vi "Set File to Run as Admin.vi"(8 "Error In":errorcluster, 11 "Path to file that needs to be run as admin":path) -> (0 "Error Out":errorcluster)   [LabVIEW 2014]
panel:
  in  "working directory":path=path ""
  out "concatenated string":string
  out "standard error":string
  out "standard output":string
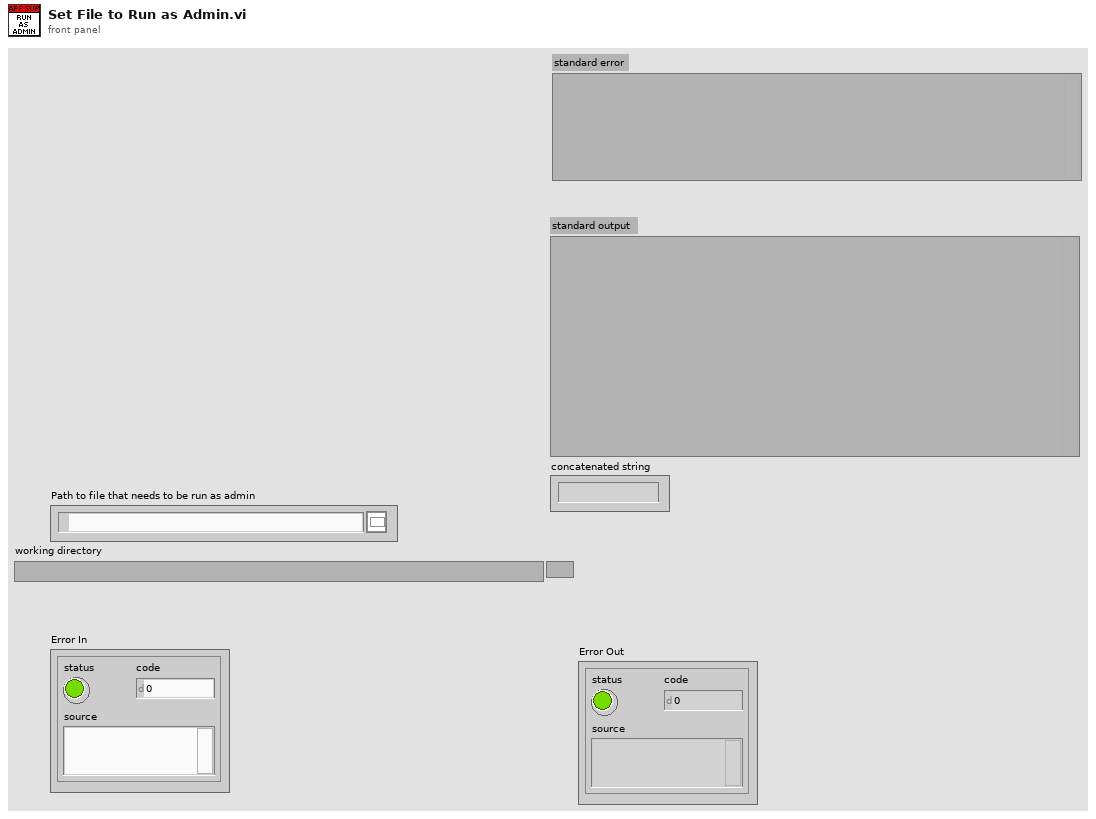
[diagram p1: front panel]
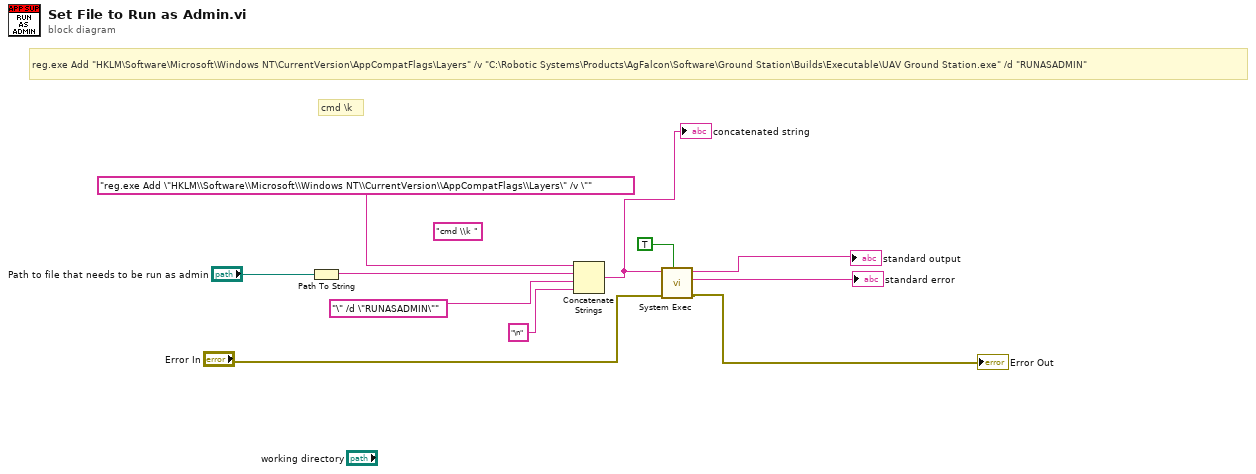
[diagram p0: block diagram]
diagram:
  (unwired) "cmd \\k " ("command line")
  # "cmd \\k"
  # "reg.exe Add \"HKLM\\Software\\Microsoft\\Windows NT\\CurrentVersion\\AppCompatFlags\\Layers\" /v \"C:\\Robotic Systems\\Products\\AgFalcon\\Software\\Ground Station\\Builds\\Executable\\UAV Ground Station.exe\" /d \"RUNASADMIN\""
  n1 = Path To String(path="Path to file that needs to be run as admin") -> (string=w9:string)
  n2 = Concatenate Strings("reg.exe Add \"HKLM\\Software\\Microsoft\\Windows NT\\CurrentVersion\\AppCompatFlags\\Layers\" /v \"" ("command line"), w9, "\" /d \"RUNASADMIN\"" ("command line"), "\n") -> (w2:string)
  "concatenated string" <- w2
  n3 = call <vilib>:"System Exec.vi"("wait until completion? (T)"=TRUE, "error in (no error)"="Error In", "command line"=w2) -> ("error out"=→"Error Out":errorcluster, "standard error"=→"standard error":string, "standard output"=→"standard output":string)  [unwired: 5 in, 1 out]
